vi "_PC_Daemon_Laser.vi"(7 "eng_mode_str":refnum<vi>, 8 "error in (no error)":errorcluster) -> (0 "error out":errorcluster)   [LabVIEW 2018]
uses:
  PublicSubVI/Ctl/RegistyFunc.ctl
  <vilib>/event_ctls.llb/eventvkey.ctl
  PublicSubVI/Class/QMH/QMH.lvclass
panel:
  in  "Laser.Current_simple":dbl(slide)=50.0 caption="Current (%)" scale=0.0..100.0
  in  "Laser.Emission_simple":bool caption="Emission"
  out "Laser.StatusString":string caption="Status"
  out "Laser Status":bool[](array[boolean])
  in  "Laser.Trigger mode":bool caption="Trigger mode"
  in  "Laser.Frequency":dbl(slide) caption="Frequency" scale=0.0..1000.0
  in  "Laser.Current":dbl(slide)=50.0 caption="Current (%)" scale=0.0..100.0
  in  "Laser.Emission":bool caption="Emission"
  out "stop":bool
  in  "mouseType":enum16{"mouseIdle", "mouseDown"}(ring)
  # "Laser Emission"
  # "Cmd Error"
  # "System Error"
  # "Standard Event"
  # "Operational"
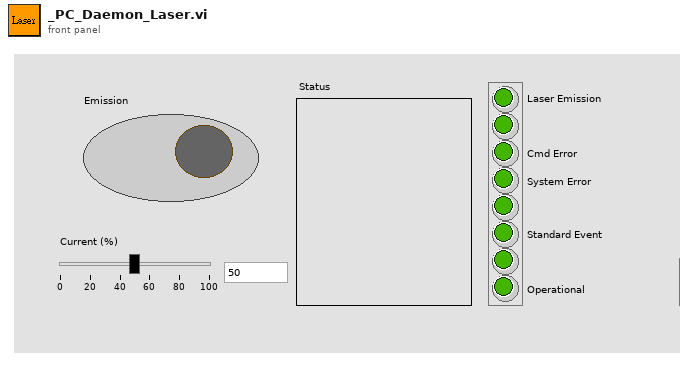
[diagram p1: front panel]
types:
  T1 = typedef "RegistyFunc.ctl" = enum16{"None", "FileAutoSave", "FileNoise", "FileSN", "ExeStatu", "WorkFolderPath", "MethodPath", "AVGItem", "LoopItem", "AutoRun", "BGColor", "LineColor", "LineWidth", "XGrid", "YGrid", "DeviceRefnum"}
  T2 = enum8{"Enabled", "Disabled", "Disabled and Grayed Out"}
  T3 = enum32{"Invalid", "Default", "Floating", "Floating/Auto-Hide", "Modal"}
  T4 = cluster{"Laser.Current":refnum<vi>, "Laser.Current_simple":refnum<vi>, "Laser.Emission":refnum<vi>, "Laser.Emission_simple":refnum<vi>, "Laser.Frequency":refnum<vi>, "Laser.Trigger mode":refnum<vi>, "Time Stamp":timestamp}
  T5 = typedef "eventvkey.ctl" = enum16{"ASCII", "Enter", "Return", "Shift", "Ctrl", "Alt", "Cmd", "Opt", "Caps", "NumLock", "Clear", "Break", "Up", "Down", "Left", "Right", "Insert", "Delete", "Home", "End", "PageUp", "PageDown", "Escape", "Help", "Pause", "ScrollLock", "F1", "F2", "F3", "F4", "F5", "F6", "F7", "F8", "F9", "F10", "F11", "F12", "F13", "F14", "F15", "F16", "F17", "F18", "F19", "F20", "F21", "F22", "F23", "F24", "Play", "VolumeUp", "VolumeDown", "Mute", "Two Byte Char"}
  T6 = typedef "_ctl_LaserParam.ctl" = cluster{"Energy":dbl, "Freq":dbl, "Emission":bool, "TriggerSource":enum16{"Internal", "External"}, "Time Stamp":timestamp}
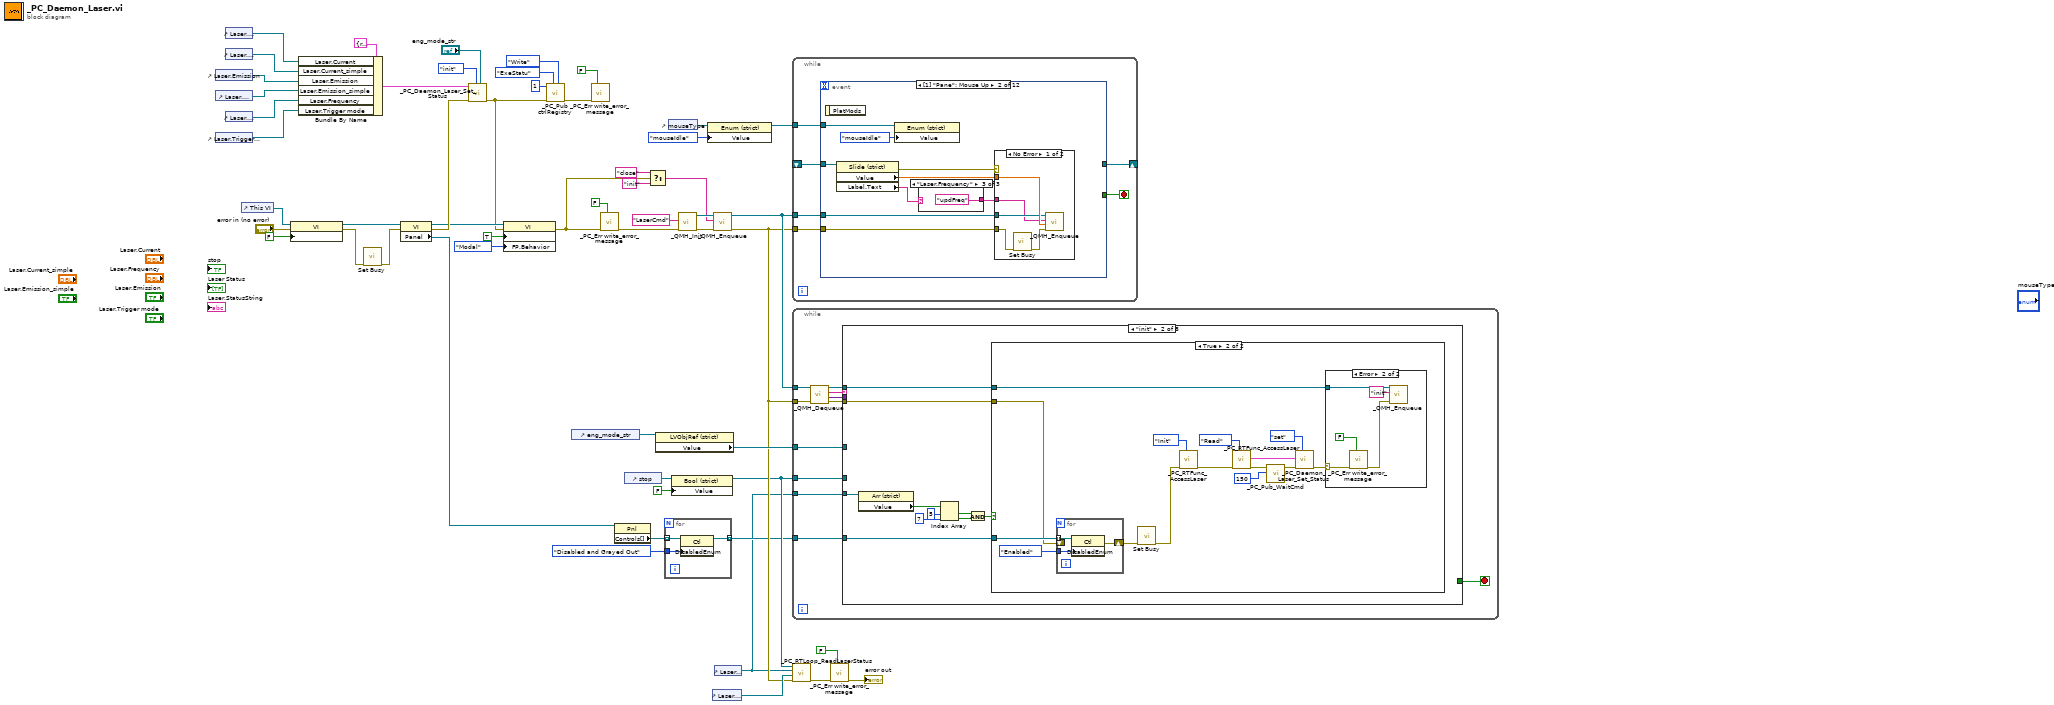
[diagram p0: block diagram]
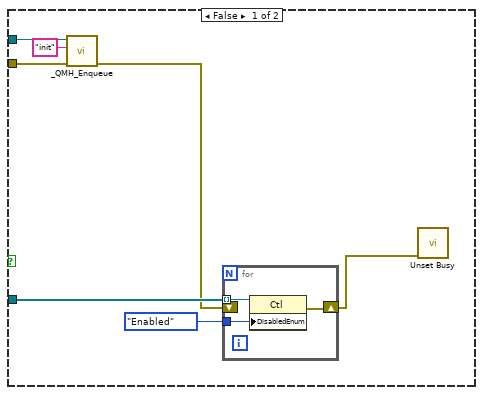
[diagram p3: hidden frame]
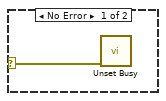
[diagram p4: hidden frame]
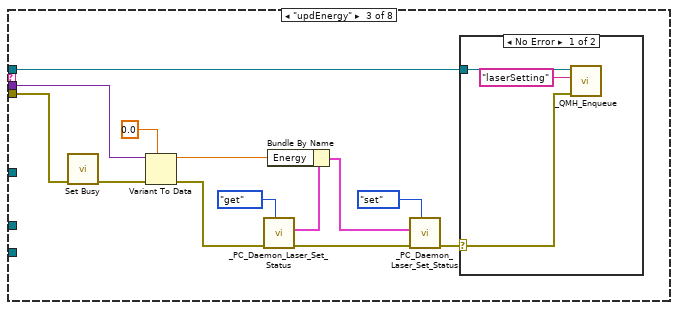
[diagram p5: hidden frame]
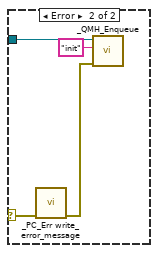
[diagram p6: hidden frame]
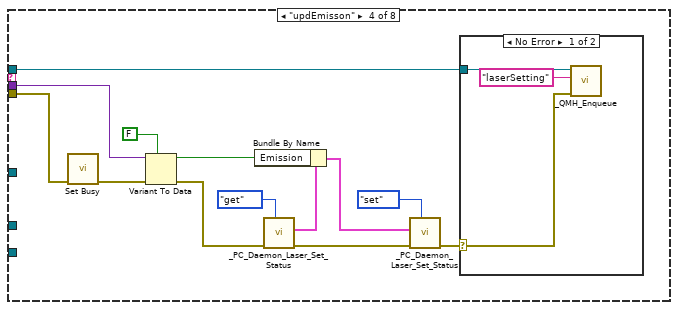
[diagram p7: hidden frame]
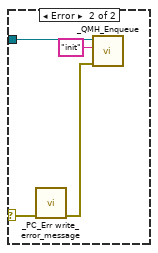
[diagram p8: hidden frame]
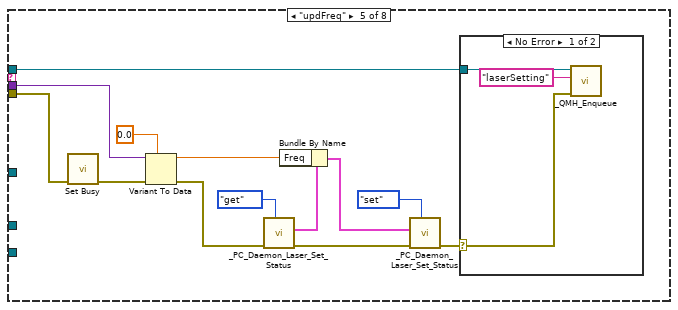
[diagram p9: hidden frame]
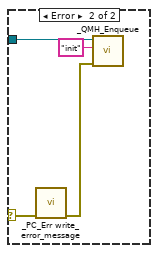
[diagram p10: hidden frame]
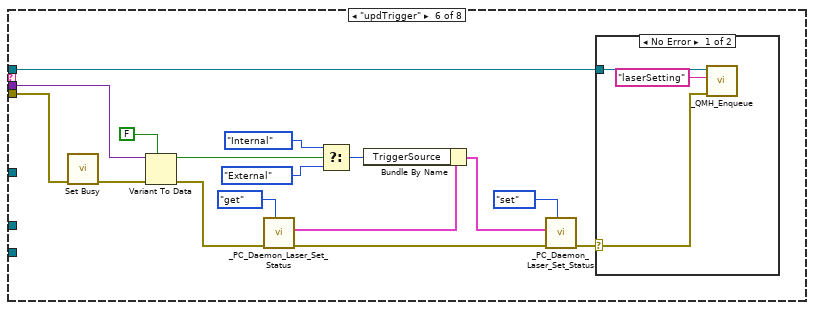
[diagram p11: hidden frame]
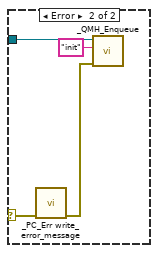
[diagram p12: hidden frame]
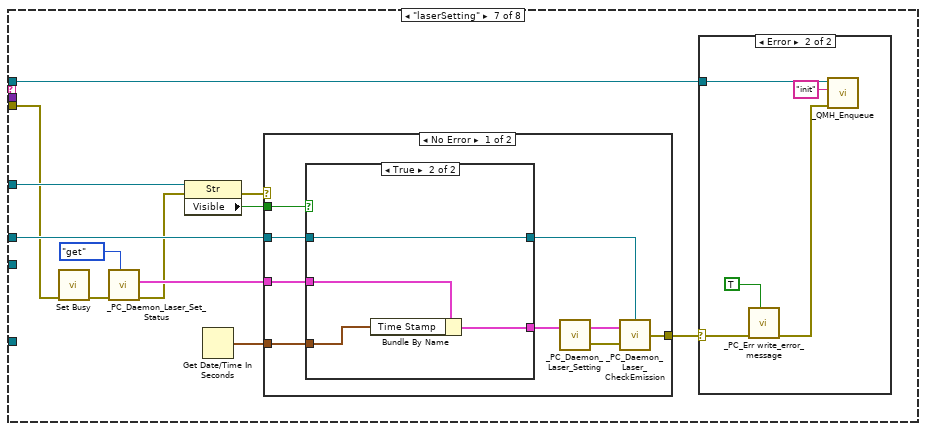
[diagram p13: hidden frame]
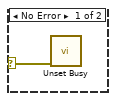
[diagram p14: hidden frame]
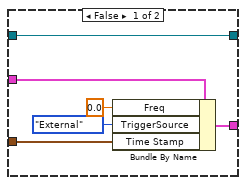
[diagram p15: hidden frame]
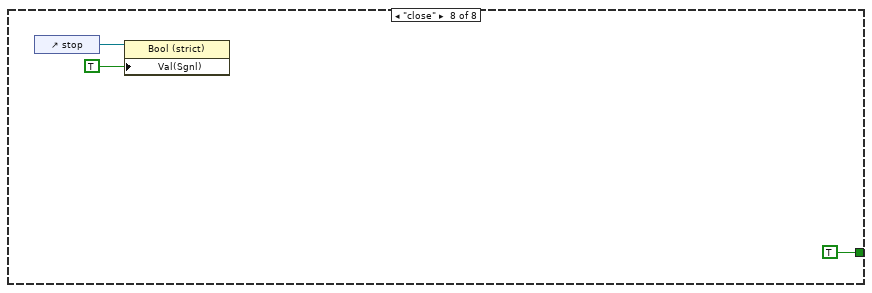
[diagram p17: hidden frame]
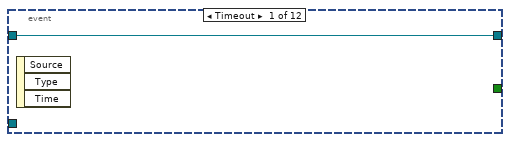
[diagram p18: hidden frame]
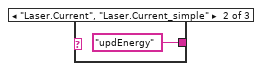
[diagram p20: hidden frame]
diagram:
  n1 = control-ref of="Laser.Emission"() -> (w38:refnum<vi>)
  n2 = control-ref of="Laser.Emission_simple"() -> (w39:refnum<vi>)
  n3 = control-ref of="Laser.Trigger mode"() -> (w41:refnum<vi>)
  n4 = control-ref of="Laser.Current"() -> (w36:refnum<vi>)
  n5 = control-ref of="Laser.Current_simple"() -> (w37:refnum<vi>)
  n6 = control-ref of="Laser.Frequency"() -> (w40:refnum<vi>)
  n7 = control-ref of="This VI"() -> (w30:refnum<vi>)
  n8 = property class="VI"(reference=w30, error in="error in (no error)", "Front Panel.IsFrontmost"=FALSE) -> (reference out=w17:refnum<vi>, error out=w8:errorcluster)
  n9 = Bundle By Name(cluster=T4 {"Laser.Current"=refnum, "Laser.Current_simple"=refnum, "Laser.Emission"=refnum, "Laser.Emission_simple"=refnum, "Laser.Frequency"=refnum, "Laser.Trigger mode"=refnum, "Time Stamp"=timestamp(0 s since 1904-01-01)} ("refnum cluster in"), "Laser.Current"=w36, "Laser.Current_simple"=w37, "Laser.Emission"=w38, "Laser.Emission_simple"=w39, "Laser.Frequency"=w40, "Laser.Trigger mode"=w41) -> (w34:T4)
  n10 = call <vilib>:"Set Busy.vi"("error in (no error)"=w8) -> ("error out"=w7:errorcluster)  [unwired: 9 in, 1 out]
  n11 = property class="VI"(reference=w17, error in=w7) -> (reference out=w10:refnum<vi>, error out=w11:errorcluster, "Panel"=w16:refnum<vi>)
  n12 = call "_PC_Daemon_Laser_Set_Status.vi"("eng_mode_str"="eng_mode_str", "function"=enum16{"none", "init", "set", "get"}."init", "error in (no error)"=w11, "refnum cluster in"=w34) -> ("error out"=w3:errorcluster)  [unwired: 6 in, 1 out]
  n13 = property class="VI"(reference=w10, error in=w3, "Front Panel.IsFrontmost"=TRUE ("Front Panel Window:Is Frontmost"), "FP.Behavior"=T3."Modal" ("Front Panel Window:Behavior")) -> (error out=w9:errorcluster)  [unwired: 1 out]
  n14 = call "_PC_Pub ctrlRegistry.vi"("type"=enum16{"None", "Write", "Read"}."Write", "function"=RegistyFunc."ExeStatu", "error in (no error)"=w3, "write value"=u32 1) -> ("error out"=w1:errorcluster)  [unwired: 4 in, 3 out]
  n15 = control-ref of="eng_mode_str"() -> (w45:refnum<vi>)
  n16 = call "_PC_Err write_error_message.vi"("show msg( T )"=FALSE, "error in"=w1) -> ()  [unwired: 9 in, 1 out]
  n17 = call "_PC_Err write_error_message.vi"("show msg( T )"=FALSE, "error in"=w9) -> ("error out"=w24:errorcluster)  [unwired: 9 in]
  n18 = property class="Pnl"(reference=w16) -> ("Controls[]"=w15:refnum<vi>[])  [unwired: 1 in, 2 out]
  n19 = control-ref of="stop"() -> (w47:refnum<vi>)
  n20 = Select(t="close" ("Msg"), s=w9, f="init" ("Msg")) -> (s? t:f=w25:string)
  n21 = property class="LVObjRef (strict)"(reference=w45) -> ("Value"=w44:refnum<vi>)  [unwired: 1 in, 2 out]
  n22 = for {
    tunnel: w15 -> [w57] mode=indexing
    tunnel: T2."Disabled and Grayed Out" ("Disabled") -> [w56]
    tunnel: [w55] -> w13 mode=indexing
    n23 = property class="Ctl"(reference=w57, "DisabledEnum"=w56) -> (reference out=w55:refnum<vi>)  [unwired: 1 in, 1 out]
  }
  n24 = control-ref of="mouseType"() -> (w54:refnum<vi>)
  n25 = property class="Bool (strict)"(reference=w47, "Value"=FALSE) -> (reference out=w19:refnum<vi>)  [unwired: 1 in, 1 out]
  n26 = call "_QMH_Init.vi"("error in (no error)"=w24, "name (unnamed)"="LaserCmd") -> ("error out"=w50:errorcluster, "QMH out"=w49:refnum<class "QMH.lvclass">)  [unwired: 8 in]
  n27 = property class="Enum (strict)"(reference=w54, "Value"=enum16{"mouseIdle", "mouseDown"}."mouseIdle") -> (reference out=w53:refnum<vi>)  [unwired: 1 in, 1 out]
  n28 = control-ref of="Laser.StatusString"() -> (w22:refnum<vi>)
  n29 = call "_QMH_Enqueue.vi"("error in (no error)"=w50, "Msg"=w25, "QMH in"=w49) -> ("error out"=w20:errorcluster, "QMH out"=w48:refnum<class "QMH.lvclass">)  [unwired: 7 in]
  n30 = control-ref of="Laser Status"() -> (w12:refnum<vi>)
  n31 = call "_PC_RTLoop_ReadLaserStatus.vi"("error in (no error)"=w20, "LaserStatus_string_reference in"=w22, "Laser Status byte"=w12, "stopRefnum"=w19) -> ("error out"=w23:errorcluster)  [unwired: 7 in]
  n32 = while {
    tunnel: w53 -> [w63]
    shift-right: [w62] -> _
    shift-left: _ -> [w61]
    tunnel: w48 -> [w60]
    tunnel: w20 -> [w59]
    stop <- w58 stop-if-true
    n33 = event shown="[1] \"Pane\": Mouse Up" {
      selector: _ -> [_ _ _ _ _ _ _ _ _ _ _ _]
      dyn-events: _ -> [_ _ _ _ _ _ _ _ _ _ _ _]
      timeout: _ -> [_ _ _ _ _ _ _ _ _ _ _ _]
      tunnel: w63 -> [_ w73 w90 w105 w107 w112 w128 _ _ _ _ _]
      tunnel: [w64 _ w85 w103 w106 w110 w123 w137 w143 w149 w151 w161] -> w62
      tunnel: w61 -> [w64 w70 w84 _ _ w109 w125 w137 w143 w149 w151 w161]
      tunnel: w60 -> [_ w69 w87 _ _ w114 w127 w142 w148 _ w154 w166]
      tunnel: w59 -> [_ w68 w86 _ _ w113 w126 w139 w145 _ w153 w163]
      tunnel: [_ _ _ _ _ _ _ _ _ w150 _ _] -> w58
      event Timeout {
        n34 = event-data() -> ()  [unwired: 1 in, 3 out]
      }
      event Mouse Up {
        n35 = event-data() -> ()  [unwired: 1 in, 1 out]
        n36 = property class="Slide (strict)"(reference=w70) -> (error out=w67:errorcluster, "Value"=w71:dbl, "Label.Text"=w66:string)  [unwired: 1 in, 1 out]
        n37 = property class="Enum (strict)"(reference=w73, "Value"=enum16{"mouseIdle", "mouseDown"}."mouseIdle") -> ()  [unwired: 1 in, 2 out]
        n38 = case shown="\"Laser.Frequency\"" w66 {
          tunnel: [_ "updEnergy" ("Msg") "updFreq" ("Msg")] -> w65
          frame "False", Default {
          }
          frame "Laser.Current", "Laser.Current_simple" {
          }
          frame "Laser.Frequency" {
          }
        }
        n39 = case shown="No Error" w67 {
          tunnel: w71 -> [w80 _]
          tunnel: w69 -> [w79 _]
          tunnel: w68 -> [w78 _]
          tunnel: w65 -> [w76 _]
          frame No Error {
            n40 = call <vilib>:"Set Busy.vi"("error in (no error)"=w78) -> ("error out"=w77:errorcluster)  [unwired: 9 in, 1 out]
            n41 = call "_QMH_Enqueue.vi"("error in (no error)"=w77, "Data"=w80, "Msg"=w76, "QMH in"=w79) -> ()  [unwired: 6 in, 2 out]
          }
          frame Error {
          }
        }
      }
      event Mouse Enter {
        n42 = event-data() -> ()  [unwired: 1 in, 1 out]
        n43 = property class="Slide (strict)"(reference=w84) -> (reference out=w83:refnum<vi>, "Value"=w82:dbl, "Label.Text"=w81:string)  [unwired: 1 in, 1 out]
        n44 = property class="Enum (strict)"(reference=w90) -> (reference out=w88:refnum<vi>, "Value"=w89:enum16{"mouseIdle", "mouseDown"})  [unwired: 1 in, 1 out]
        n45 = case shown="\"mouseDown\"" w89 {
          tunnel: w88 -> [_ w100]
          tunnel: w83 -> [w91 w95]
          tunnel: w87 -> [_ w98]
          tunnel: w86 -> [_ w96]
          tunnel: [w91 w95] -> w85
          tunnel: w82 -> [_ w94]
          tunnel: w81 -> [_ w92]
          frame "mouseIdle", Default {
          }
          frame "mouseDown" {
            n46 = case shown="\"Laser.Frequency\"" w92 {
              tunnel: [_ "updEnergy" ("Msg") "updFreq" ("Msg")] -> w93
              frame "False", Default {
              }
              frame "Laser.Current", "Laser.Current_simple" {
              }
              frame "Laser.Frequency" {
              }
            }
            n47 = property class="Enum (strict)"(reference=w100, "Value"=enum16{"mouseIdle", "mouseDown"}."mouseIdle") -> ()  [unwired: 1 in, 2 out]
            n48 = call <vilib>:"Set Busy.vi"("error in (no error)"=w96) -> ("error out"=w97:errorcluster)  [unwired: 9 in, 1 out]
            n49 = call "_QMH_Enqueue.vi"("error in (no error)"=w97, "Data"=w94, "Msg"=w93, "QMH in"=w98) -> ()  [unwired: 6 in, 2 out]
          }
        }
      }
      event "Laser.Current", "Laser.Current_simple": Mouse Down? {
        n50 = event-data() -> ("CtlRef"=w103:refnum<vi>)  [unwired: 1 in]
        n51 = property class="Enum (strict)"(reference=w105, "Value"=enum16{"mouseIdle", "mouseDown"}."mouseDown") -> ()  [unwired: 1 in, 2 out]
        n52 = event-data() -> ()  [unwired: 2 in, 1 out]
      }
      event "Laser.Frequency": Mouse Down? {
        n53 = event-data() -> ("CtlRef"=w106:refnum<vi>)  [unwired: 1 in]
        n54 = property class="Enum (strict)"(reference=w107, "Value"=enum16{"mouseIdle", "mouseDown"}."mouseDown") -> ()  [unwired: 1 in, 2 out]
        n55 = event-data() -> ()  [unwired: 2 in, 1 out]
      }
      event "Laser.Current_simple", "Laser.Current": Value Change {
        n56 = event-data() -> ("NewVal"=w115:dbl)  [unwired: 1 in]
        n57 = property class="Enum (strict)"(reference=w112) -> ("Value"=w111:enum16{"mouseIdle", "mouseDown"})  [unwired: 1 in, 2 out]
        n58 = case shown="\"mouseIdle\", Default" w111 {
          tunnel: w115 -> [w121 _]
          tunnel: w114 -> [w120 _]
          tunnel: w113 -> [w119 _]
          tunnel: [w116 w122] -> w110
          tunnel: w109 -> [w116 w122]
          frame "mouseIdle", Default {
            n59 = call <vilib>:"Set Busy.vi"("error in (no error)"=w119) -> ("error out"=w117:errorcluster)  [unwired: 9 in, 1 out]
            n60 = call "_QMH_Enqueue.vi"("error in (no error)"=w117, "Data"=w121, "Msg"="updEnergy", "QMH in"=w120) -> ()  [unwired: 6 in, 2 out]
          }
          frame "mouseDown" {
          }
        }
      }
      event "Laser.Frequency": Value Change {
        n61 = event-data() -> ("NewVal"=w124:dbl)  [unwired: 1 in]
        n62 = property class="Enum (strict)"(reference=w128) -> ("Value"=w129:enum16{"mouseIdle", "mouseDown"})  [unwired: 1 in, 2 out]
        n63 = case shown="\"mouseIdle\", Default" w129 {
          tunnel: w124 -> [w135 _]
          tunnel: w127 -> [w134 _]
          tunnel: w126 -> [w133 _]
          tunnel: [w130 w136] -> w123
          tunnel: w125 -> [w130 w136]
          frame "mouseIdle", Default {
            n64 = call <vilib>:"Set Busy.vi"("error in (no error)"=w133) -> ("error out"=w131:errorcluster)  [unwired: 9 in, 1 out]
            n65 = call "_QMH_Enqueue.vi"("error in (no error)"=w131, "Data"=w135, "Msg"="updFreq", "QMH in"=w134) -> ()  [unwired: 6 in, 2 out]
          }
          frame "mouseDown" {
          }
        }
      }
      event "Laser.Emission", "Laser.Emission_simple": Value Change {
        n66 = event-data() -> ("NewVal"=w140:bool)  [unwired: 1 in]
        n67 = call <vilib>:"Set Busy.vi"("error in (no error)"=w139) -> ("error out"=w138:errorcluster)  [unwired: 9 in, 1 out]
        n68 = call "_QMH_Enqueue.vi"("error in (no error)"=w138, "Data"=w140, "Msg"="updEmisson", "QMH in"=w142) -> ()  [unwired: 6 in, 2 out]
      }
      event "Laser.Trigger mode": Value Change {
        n69 = event-data() -> ("NewVal"=w147:bool)  [unwired: 1 in]
        n70 = call <vilib>:"Set Busy.vi"("error in (no error)"=w145) -> ("error out"=w144:errorcluster)  [unwired: 9 in, 1 out]
        n71 = call "_QMH_Enqueue.vi"("error in (no error)"=w144, "Data"=w147, "Msg"="updTrigger", "QMH in"=w148) -> ()  [unwired: 6 in, 2 out]
      }
      event "stop": Value Change {
        n72 = event-data() -> ("NewVal"=w150:bool)  [unwired: 1 in]
      }
      event Key Down? {
        n73 = event-data() -> ("VKey"=w155:T5)  [unwired: 1 in]
        n74 = Equal?(x=w155, y=eventvkey."Escape") -> (x = y?=w152:bool)
        n75 = case shown="True" w152 {
          tunnel: w154 -> [_ w159]
          tunnel: w153 -> [_ w158]
          frame False {
          }
          frame True {
            n76 = call <vilib>:"Set Busy.vi"("error in (no error)"=w158) -> ("error out"=w157:errorcluster)  [unwired: 9 in, 1 out]
            n77 = call "_QMH_Enqueue.vi"("error in (no error)"=w157, "Msg"="close", "QMH in"=w159) -> ()  [unwired: 7 in, 2 out]
          }
        }
        n78 = event-data("Discard?"=w152) -> ()  [unwired: 1 in, 1 out]
      }
      event Panel Close? {
        n79 = event-data() -> ()  [unwired: 1 in, 1 out]
        n80 = call <vilib>:"Set Busy.vi"("error in (no error)"=w163) -> ("error out"=w162:errorcluster)  [unwired: 9 in, 1 out]
        n81 = call "_QMH_Enqueue.vi"("error in (no error)"=w162, "Msg"="close", "QMH in"=w166) -> ()  [unwired: 7 in, 2 out]
        n82 = event-data("Discard?"=TRUE) -> ()  [unwired: 1 in, 1 out]
      }
    }
  }
  n83 = while {
    tunnel: w48 -> [w177]
    tunnel: w20 -> [w176]
    tunnel: w19 -> [w171]
    tunnel: w44 -> [w170]
    tunnel: w13 -> [w168]
    tunnel: w12 -> [w167]
    stop <- w169 stop-if-true
    n84 = call "_QMH_Dequeue.vi"("error in (no error)"=w176, "QMH in"=w177) -> ("error out"=w173:errorcluster, "Data"=w172:variant, "Msg"=w175:string, "QMH out"=w174:refnum<class "QMH.lvclass">)  [unwired: 4 in, 2 out]
    n85 = case shown="\"init\"" w175 {
      tunnel: w174 -> [_ w186 w225 w246 w266 w292 w307 _]
      tunnel: w173 -> [_ w187 w224 w245 w265 w291 w306 _]
      tunnel: w172 -> [_ _ w232 w252 w272 w295 _ _]
      tunnel: w171 -> [_ _ _ _ _ _ w312 _]
      tunnel: w170 -> [_ _ _ _ _ _ w315 _]
      tunnel: [_ _ _ _ _ _ _ TRUE] -> w169
      tunnel: w168 -> [_ w179 _ _ _ _ _ _]
      tunnel: w167 -> [_ w181 _ _ _ _ _ _]
      frame Default {
      }
      frame "init" {
        n86 = property class="Arr (strict)"(reference=w181) -> ("Value"=w178:bool[])  [unwired: 1 in, 2 out]
        n87 = Index Array(array=w178, index #1=5 ("index"), index #2=7 ("index")) -> (element #1=w183:bool, element #2=w182:bool)
        n88 = And(x=w183, y=w182) -> (x .and. y?=w180:bool)
        n89 = case shown="True" w180 {
          tunnel: w187 -> [w192 w199]
          tunnel: w186 -> [w193 w202]
          tunnel: w179 -> [w190 w201]
          frame False {
            n90 = call "_QMH_Enqueue.vi"("error in (no error)"=w192, "Msg"="init", "QMH in"=w193) -> ("error out"=w189:errorcluster)  [unwired: 7 in, 1 out]
            n91 = for {
              tunnel: w190 -> [w197] mode=indexing
              tunnel: T2."Enabled" ("Disabled") -> [w196]
              shift-right: [w195] -> w188
              shift-left: w189 -> [_]
              n92 = property class="Ctl"(reference=w197, "DisabledEnum"=w196) -> (error out=w195:errorcluster)  [unwired: 1 in, 1 out]
            }
            n93 = call <vilib>:"Unset Busy.vi"("error in (no error)"=w188) -> ()  [unwired: 10 in, 1 out]
          }
          frame True {
            n94 = for {
              tunnel: w201 -> [w215] mode=indexing
              tunnel: T2."Enabled" ("Disabled") -> [w214]
              shift-right: [w213] -> w198
              shift-left: w199 -> [_]
              n95 = property class="Ctl"(reference=w215, "DisabledEnum"=w214) -> (error out=w213:errorcluster)  [unwired: 1 in, 1 out]
            }
            n96 = call <vilib>:"Set Busy.vi"("error in (no error)"=w198) -> ("error out"=w210:errorcluster)  [unwired: 9 in, 1 out]
            n97 = call "_PC_RTFunc_AccessLaser.vi"("Function"=enum16{"Init", "Write", "Read"}."Init", "error in (no error)"=w210) -> ("error out"=w206:errorcluster)  [unwired: 8 in, 1 out]
            n98 = call "_PC_RTFunc_AccessLaser.vi"("Function"=enum16{"Init", "Write", "Read"}."Read", "error in (no error)"=w206) -> ("error out"=w205:errorcluster, "LaserSetting"=w212:T6)  [unwired: 8 in]
            n99 = call "_PC_Pub_WaitCmd.vi"("milliseconds to wait"=u32 150, "error in (no error)"=w205) -> ("error out"=w211:errorcluster)  [unwired: 9 in]
            n100 = call "_PC_Daemon_Laser_Set_Status.vi"("function"=enum16{"none", "init", "set", "get"}."set", "error in (no error)"=w211, "LaserSetting in"=w212) -> ("error out"=w203:errorcluster)  [unwired: 7 in, 1 out]
            n101 = case shown="Error" w203 {
              selector: w203 -> [w216 w219]
              tunnel: w202 -> [_ w220]
              frame No Error {
                n102 = call <vilib>:"Unset Busy.vi"("error in (no error)"=w216) -> ()  [unwired: 10 in, 1 out]
              }
              frame Error {
                n103 = call "_PC_Err write_error_message.vi"("show msg( T )"=FALSE, "error in"=w219) -> ("error out"=w217:errorcluster)  [unwired: 9 in]
                n104 = call "_QMH_Enqueue.vi"("error in (no error)"=w217, "Msg"="init", "QMH in"=w220) -> ()  [unwired: 7 in, 2 out]
              }
            }
          }
        }
      }
      frame "updEnergy" {
        n105 = call <vilib>:"Set Busy.vi"("error in (no error)"=w224) -> ("error out"=w223:errorcluster)  [unwired: 9 in, 1 out]
        n106 = Variant To Data(error in=w223, type=0.0 ("Value"), Variant=w232) -> (data=w228:dbl, error out=w230:errorcluster)
        n107 = call "_PC_Daemon_Laser_Set_Status.vi"("function"=enum16{"none", "init", "set", "get"}."get", "error in (no error)"=w230) -> ("error out"=w226:errorcluster, "LaserSetting out"=w229:T6)  [unwired: 8 in]
        n108 = Bundle By Name(cluster=w229, "Energy"=w228) -> (w227:T6)
        n109 = call "_PC_Daemon_Laser_Set_Status.vi"("function"=enum16{"none", "init", "set", "get"}."set", "error in (no error)"=w226, "LaserSetting in"=w227) -> ("error out"=w222:errorcluster)  [unwired: 7 in, 1 out]
        n110 = case shown="No Error" w222 {
          selector: w222 -> [w235 w241]
          tunnel: w225 -> [w236 w239]
          frame No Error {
            n111 = call "_QMH_Enqueue.vi"("error in (no error)"=w235, "Msg"="laserSetting", "QMH in"=w236) -> ()  [unwired: 7 in, 2 out]
          }
          frame Error {
            n112 = call "_PC_Err write_error_message.vi"("error in"=w241) -> ("error out"=w238:errorcluster)  [unwired: 10 in]
            n113 = call "_QMH_Enqueue.vi"("error in (no error)"=w238, "Msg"="init", "QMH in"=w239) -> ()  [unwired: 7 in, 2 out]
          }
        }
      }
      frame "updEmisson" {
        n114 = call <vilib>:"Set Busy.vi"("error in (no error)"=w245) -> ("error out"=w244:errorcluster)  [unwired: 9 in, 1 out]
        n115 = Variant To Data(error in=w244, type=FALSE, Variant=w252) -> (data=w249:bool, error out=w251:errorcluster)
        n116 = call "_PC_Daemon_Laser_Set_Status.vi"("function"=enum16{"none", "init", "set", "get"}."get", "error in (no error)"=w251) -> ("error out"=w247:errorcluster, "LaserSetting out"=w250:T6)  [unwired: 8 in]
        n117 = Bundle By Name(cluster=w250, "Emission"=w249) -> (w248:T6)
        n118 = call "_PC_Daemon_Laser_Set_Status.vi"("function"=enum16{"none", "init", "set", "get"}."set", "error in (no error)"=w247, "LaserSetting in"=w248) -> ("error out"=w243:errorcluster)  [unwired: 7 in, 1 out]
        n119 = case shown="No Error" w243 {
          selector: w243 -> [w255 w261]
          tunnel: w246 -> [w256 w259]
          frame No Error {
            n120 = call "_QMH_Enqueue.vi"("error in (no error)"=w255, "Msg"="laserSetting", "QMH in"=w256) -> ()  [unwired: 7 in, 2 out]
          }
          frame Error {
            n121 = call "_PC_Err write_error_message.vi"("error in"=w261) -> ("error out"=w258:errorcluster)  [unwired: 10 in]
            n122 = call "_QMH_Enqueue.vi"("error in (no error)"=w258, "Msg"="init", "QMH in"=w259) -> ()  [unwired: 7 in, 2 out]
          }
        }
      }
      frame "updFreq" {
        n123 = call <vilib>:"Set Busy.vi"("error in (no error)"=w265) -> ("error out"=w264:errorcluster)  [unwired: 9 in, 1 out]
        n124 = Variant To Data(error in=w264, type=0.0, Variant=w272) -> (data=w269:dbl, error out=w271:errorcluster)
        n125 = call "_PC_Daemon_Laser_Set_Status.vi"("function"=enum16{"none", "init", "set", "get"}."get", "error in (no error)"=w271) -> ("error out"=w267:errorcluster, "LaserSetting out"=w270:T6)  [unwired: 8 in]
        n126 = Bundle By Name(cluster=w270, "Freq"=w269) -> (w268:T6)
        n127 = call "_PC_Daemon_Laser_Set_Status.vi"("function"=enum16{"none", "init", "set", "get"}."set", "error in (no error)"=w267, "LaserSetting in"=w268) -> ("error out"=w263:errorcluster)  [unwired: 7 in, 1 out]
        n128 = case shown="No Error" w263 {
          selector: w263 -> [w275 w281]
          tunnel: w266 -> [w276 w279]
          frame No Error {
            n129 = call "_QMH_Enqueue.vi"("error in (no error)"=w275, "Msg"="laserSetting", "QMH in"=w276) -> ()  [unwired: 7 in, 2 out]
          }
          frame Error {
            n130 = call "_PC_Err write_error_message.vi"("error in"=w281) -> ("error out"=w278:errorcluster)  [unwired: 10 in]
            n131 = call "_QMH_Enqueue.vi"("error in (no error)"=w278, "Msg"="init", "QMH in"=w279) -> ()  [unwired: 7 in, 2 out]
          }
        }
      }
      frame "updTrigger" {
        n132 = call <vilib>:"Set Busy.vi"("error in (no error)"=w291) -> ("error out"=w290:errorcluster)  [unwired: 9 in, 1 out]
        n133 = Variant To Data(error in=w290, type=FALSE, Variant=w295) -> (data=w282:bool, error out=w294:errorcluster)
        n134 = call "_PC_Daemon_Laser_Set_Status.vi"("function"=enum16{"none", "init", "set", "get"}."get", "error in (no error)"=w294) -> ("error out"=w293:errorcluster, "LaserSetting out"=w283:T6)  [unwired: 8 in]
        n135 = Select(t=enum16{"Internal", "External"}."Internal" ("TriggerSource"), s=w282, f=enum16{"Internal", "External"}."External" ("TriggerSource")) -> (s? t:f=w285:enum16{"Internal", "External"})
        n136 = Bundle By Name(cluster=w283, "TriggerSource"=w285) -> (w284:T6)
        n137 = call "_PC_Daemon_Laser_Set_Status.vi"("function"=enum16{"none", "init", "set", "get"}."set", "error in (no error)"=w293, "LaserSetting in"=w284) -> ("error out"=w289:errorcluster)  [unwired: 7 in, 1 out]
        n138 = case shown="No Error" w289 {
          selector: w289 -> [w298 w304]
          tunnel: w292 -> [w299 w302]
          frame No Error {
            n139 = call "_QMH_Enqueue.vi"("error in (no error)"=w298, "Msg"="laserSetting", "QMH in"=w299) -> ()  [unwired: 7 in, 2 out]
          }
          frame Error {
            n140 = call "_PC_Err write_error_message.vi"("error in"=w304) -> ("error out"=w301:errorcluster)  [unwired: 10 in]
            n141 = call "_QMH_Enqueue.vi"("error in (no error)"=w301, "Msg"="init", "QMH in"=w302) -> ()  [unwired: 7 in, 2 out]
          }
        }
      }
      frame "laserSetting" {
        n142 = call <vilib>:"Set Busy.vi"("error in (no error)"=w306) -> ("error out"=w305:errorcluster)  [unwired: 9 in, 1 out]
        n143 = call "_PC_Daemon_Laser_Set_Status.vi"("function"=enum16{"none", "init", "set", "get"}."get", "error in (no error)"=w305) -> ("error out"=w310:errorcluster, "LaserSetting out"=w313:T6)  [unwired: 8 in]
        n144 = property class="Str"(reference=w315, error in=w310) -> (error out=w309:errorcluster, "Visible"=w314:bool)  [unwired: 1 out]
        n145 = Get Date/Time In Seconds() -> (seconds since 1Jan1904=w311:timestamp)
        n146 = case shown="No Error" w309 {
          selector: w309 -> [_ w342]
          tunnel: w314 -> [w331 _]
          tunnel: w313 -> [w330 _]
          tunnel: w312 -> [w329 _]
          tunnel: w311 -> [w328 _]
          tunnel: [w324 w342] -> w308
          frame No Error {
            n147 = case shown="True" w331 {
              tunnel: w330 -> [w337 w340]
              tunnel: w329 -> [w336 w341]
              tunnel: [w336 w341] -> w325
              tunnel: w328 -> [w335 w339]
              tunnel: [w332 w338] -> w326
              frame False {
                n148 = Bundle By Name(cluster=w337, "Freq"=0.0, "TriggerSource"=enum16{"Internal", "External"}."External", "Time Stamp"=w335) -> (w332:T6)
              }
              frame True {
                n149 = Bundle By Name(cluster=w340, "Time Stamp"=w339) -> (w338:T6)
              }
            }
            n150 = call "_PC_Daemon_Laser_Setting.vi"("Data"=w326) -> ("error out"=w327:errorcluster, "LaserSetting"=w323:T6)  [unwired: 1 in]
            n151 = call "_PC_Daemon_Laser_CheckEmission.vi"("stopRefnum"=w325, "error in (no error)"=w327, "_cluster_Laser349"=w323) -> ("error out"=w324:errorcluster)
          }
          frame Error {
          }
        }
        n152 = case shown="Error" w308 {
          selector: w308 -> [w317 w320]
          tunnel: w307 -> [_ w322]
          frame No Error {
            n153 = call <vilib>:"Unset Busy.vi"("error in (no error)"=w317) -> ()  [unwired: 10 in, 1 out]
          }
          frame Error {
            n154 = call "_PC_Err write_error_message.vi"("show msg( T )"=TRUE, "error in"=w320) -> ("error out"=w318:errorcluster)  [unwired: 9 in]
            n155 = call "_QMH_Enqueue.vi"("error in (no error)"=w318, "Msg"="init", "QMH in"=w322) -> ()  [unwired: 7 in, 2 out]
          }
        }
      }
      frame "close" {
        n156 = control-ref of="stop"() -> (w344:refnum<vi>)
        n157 = property class="Bool (strict)"(reference=w344, "Val(Sgnl)"=TRUE ("Value (Signaling)")) -> ()  [unwired: 1 in, 2 out]
      }
    }
  }
  n158 = call "_PC_Err write_error_message.vi"("show msg( T )"=FALSE, "error in"=w23) -> ("error out"=→"error out":errorcluster)  [unwired: 9 in]
